vi "First Step.vi"(8 "error in (no error)":errorcluster, 11 "Pulse Gen Basic Scan.lvclass in":refnum<class "Pulse Gen Basic Scan.lvclass">) -> (0 "error out":errorcluster, 2 "Current Position":dbl, 3 "Pulse Gen Basic Scan.lvclass out":refnum<class "Pulse Gen Basic Scan.lvclass">)   [LabVIEW 2009, in "Pulse Gen Basic Scan.lvclass"]
doc: "(Dynamic) Reset the instrument and prepare to scan. Go to step #0 - the first step. If desired, the scanner may do this in a different way than usual (i.e. by preparing to move a long distance, or reset to home position.)"
uses:
  Pulse Gen Basic Scan.lvclass
  Scanner/Scanner.lvclass
  Instruments/Utility Classes/Scannable/Scannable.lvclass
  Pulse Gen Basic Scan.lvclass/Pulse Gen Basic Scan.ctl
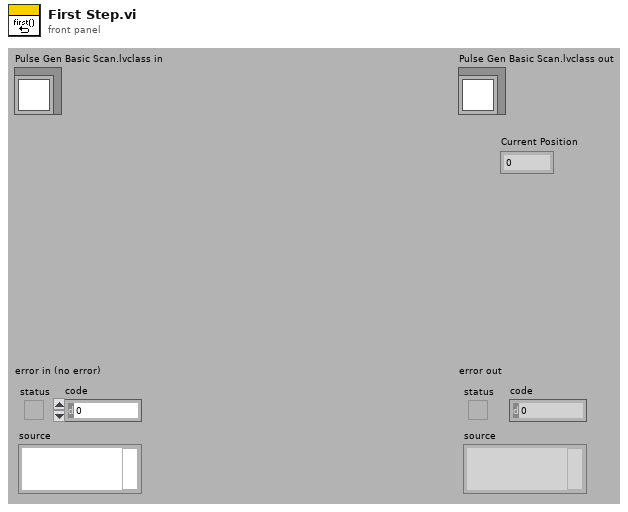
[diagram p1: front panel]
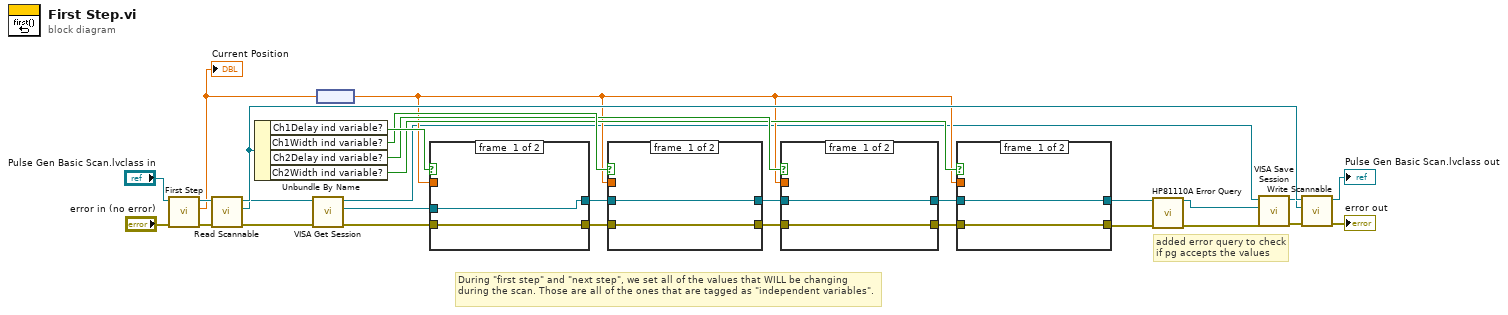
[diagram p0: block diagram]
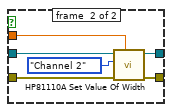
[diagram p2: hidden frame]
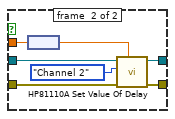
[diagram p3: hidden frame]
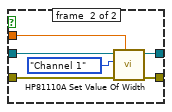
[diagram p4: hidden frame]
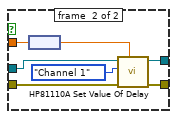
[diagram p5: hidden frame]
diagram:
  # "added error query to check\nif pg accepts the values"
  # "During \"first step\" and \"next step\", we set all of the values that WILL be changing during the scan. Those are all of the ones that are tagged as \"independent variables\"."
  n1 = call-parent "First Step.vi"("error in (no error)"="error in (no error)", "Scanner.lvclass in"="Pulse Gen Basic Scan.lvclass in") -> ("error out"=w15:errorcluster, "Current Position"=w8:dbl, "Scanner.lvclass out"=w18:refnum<class "Pulse Gen Basic Scan.lvclass">)  [unwired: 7 in]
  "Current Position" <- w8
  n2 = call-dynamic "Read Scannable.vi"("error in (no error)"=w15, "Scanner.lvclass in"=w18) -> ("error out"=w14:errorcluster, "Scannable.lvclass"=w12:refnum<class "Scannable.lvclass">, "Scanner.lvclass out"=w17:refnum<class "Pulse Gen Basic Scan.lvclass">)  [unwired: 7 out]
  n3 = Unbundle By Name(w17) -> ("Ch1Delay ind variable?"=w22:bool, "Ch1Width ind variable?"=w21:bool, "Ch2Delay ind variable?"=w20:bool, "Ch2Width ind variable?"=w19:bool)
  n4 = call-dynamic "VISA Get Session.vi"("error in (no error)"=w14, "Instrument.lvclass in"=w12) -> ("error out"=w13:errorcluster, "VISA Resource Name"=w6:refnum<visa-resource-name>, "Instrument.lvclass out"=w5:refnum<class "Scannable.lvclass">)  [unwired: 7 out]
  n5 = node(w8) -> (w7:dbl[unit])
  n6 = case shown="True" w22 {
    tunnel: [w31 w39] -> w28
    tunnel: w13 -> [w32 w38]
    tunnel: [w32 w37] -> w25
    tunnel: w7 -> [_ w35]
    tunnel: w6 -> [w31 w33]
    frame #0 {
    }
    frame #1 {
      n7 = node(w35) -> (w34:dbl)
      n8 = call "HP81110A Set Value Of Delay.vi"("Delay Value (0.0)"=w34, "error in (no error)"=w38, "Channel (1:Channel 1)"=enum16{"Channel All ", "Channel 1", "Channel 2"}."Channel 1", "VISA session"=w33) -> ("error out"=w37:errorcluster, "dup VISA session"=w39:refnum<visa-resource-name>)  [unwired: 6 in]
    }
  }
  n9 = case shown="True" w21 {
    tunnel: w28 -> [w41 w47]
    tunnel: [w41 w46] -> w27
    tunnel: w25 -> [w40 w45]
    tunnel: [w40 w44] -> w24
    tunnel: w7 -> [_ w42]
    frame #0 {
    }
    frame #1 {
      n10 = call "HP81110A Set Value Of Width.vi"("Width Value (100.0E-9)"=w42, "error in (no error)"=w45, "Channel (1:Channel 1)"=enum16{"Channel All ", "Channel 1", "Channel 2"}."Channel 1", "VISA session"=w47) -> ("error out"=w44:errorcluster, "dup VISA session"=w46:refnum<visa-resource-name>)  [unwired: 6 in]
    }
  }
  n11 = case shown="True" w20 {
    tunnel: w27 -> [w49 w56]
    tunnel: [w49 w55] -> w26
    tunnel: w24 -> [w48 w54]
    tunnel: [w48 w53] -> w23
    tunnel: w7 -> [_ w51]
    frame #0 {
    }
    frame #1 {
      n12 = node(w51) -> (w50:dbl)
      n13 = call "HP81110A Set Value Of Delay.vi"("Delay Value (0.0)"=w50, "error in (no error)"=w54, "Channel (1:Channel 1)"=enum16{"Channel All ", "Channel 1", "Channel 2"}."Channel 2", "VISA session"=w56) -> ("error out"=w53:errorcluster, "dup VISA session"=w55:refnum<visa-resource-name>)  [unwired: 6 in]
    }
  }
  n14 = case shown="True" w19 {
    tunnel: w26 -> [w57 w64]
    tunnel: w23 -> [w58 w63]
    tunnel: [w58 w62] -> w4
    tunnel: w7 -> [_ w60]
    tunnel: [w57 w59] -> w3
    frame #0 {
    }
    frame #1 {
      n15 = call "HP81110A Set Value Of Width.vi"("Width Value (100.0E-9)"=w60, "error in (no error)"=w63, "Channel (1:Channel 1)"=enum16{"Channel All ", "Channel 1", "Channel 2"}."Channel 2", "VISA session"=w64) -> ("error out"=w62:errorcluster, "dup VISA session"=w59:refnum<visa-resource-name>)  [unwired: 6 in]
    }
  }
  n16 = call "HP81110A Error Query.vi"("VISA session"=w3, "error in (no error)"=w4) -> ("dup VISA session"=w2:refnum<visa-resource-name>, "error out"=w1:errorcluster)  [unwired: 10 in, 2 out]
  n17 = call-dynamic "VISA Save Session.vi"("error in (no error)"=w1, "VISA Resource Name"=w2, "Instrument.lvclass in"=w5) -> ("error out"=w10:errorcluster, "Instrument.lvclass out"=w11:refnum<class "Scannable.lvclass">)  [unwired: 7 out]
  n18 = call-dynamic "Write Scannable.vi"("error in (no error)"=w10, "Scannable.lvclass"=w11, "Scanner.lvclass in"=w17) -> ("error out"=→"error out":errorcluster, "Scanner.lvclass out"=→"Pulse Gen Basic Scan.lvclass out":refnum<class "Pulse Gen Basic Scan.lvclass">)  [unwired: 7 out]
